vi "MetaServer.vi"(6 "Pause/Stop":cluster{"Exp Stop":bool, "ExpRun 2":bool}, 10 "File Paths":T1={"Local Save Path"=path "\\\\smbhome.uscs.susx.ac.uk\\cv222/Desktop/data", "Newton Save Path"=path "Z:/#Projects/Entanglement/data", "File Name"="test", "LocalSave"=TRUE}, 11 "Compiler Settings":T2={"Python Path"=path "", "Main File"="makesequence.py", "Meta File"="makesequence.py", "Aux File"="makesequence.py"}) -> ()   [LabVIEW 2017]
uses:
  PulseCompiler/CompilerSettings.ctl
  controls/FilePaths.ctl
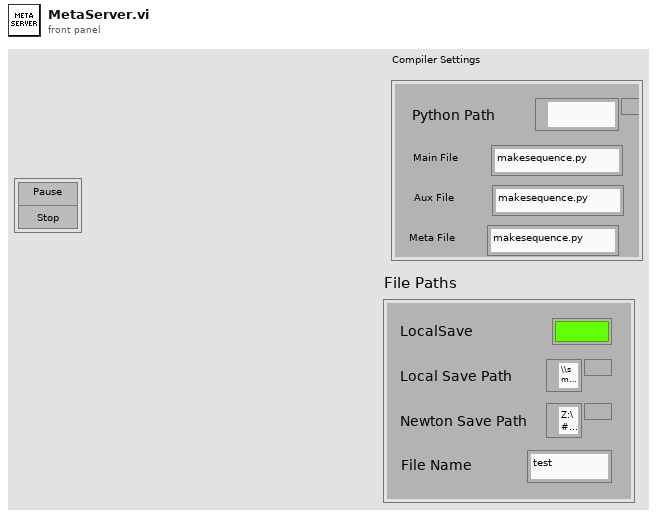
[diagram p1: front panel]
types:
  T1 = typedef "FilePaths.ctl" = cluster{"Local Save Path":path, "Newton Save Path":path, "File Name":string, "LocalSave":bool}
  T2 = typedef "CompilerSettings.ctl" = cluster{"Python Path":path, "Main File":string, "Meta File":string, "Aux File":string}
  T3 = cluster{"command":string, "steps":i32, "runs":i32}[]
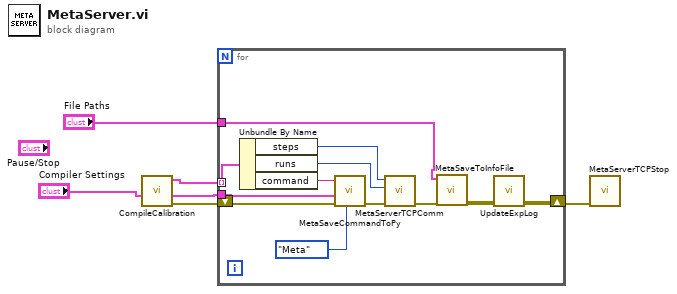
[diagram p0: block diagram]
diagram:
  n1 = call "CompileCalibration.vi"("Compiler Settings"="Compiler Settings") -> ("error out"=w5:errorcluster, "Compiler Settings 2"=w4:T2, "Exp out"=w6:T3)  [unwired: 8 in]
  n2 = for {
    tunnel: w6 -> [w18] mode=indexing
    tunnel: w4 -> [w14]
    shift-right: [w7] -> w2
    shift-left: w5 -> [w15]
    tunnel: "File Paths" -> [w11]
    n3 = Unbundle By Name(w18) -> ("steps"=w13:i32, "runs"=w12:i32, "command"=w17:string)
    n4 = call "MetaSaveCommandToPy.vi"("MetaorMain"=enum16{"Meta", "Main"}."Meta", "error in"=w15, "Compiler Settings In"=w14, "command"=w17) -> ("error out"=w10:errorcluster)  [unwired: 6 in, 1 out]
    n5 = call "MetaServerTCPComm.vi"("error in (no error)"=w10, "runs"=w12, "steps"=w13) -> ("error out"=w9:errorcluster)  [unwired: 8 in]
    n6 = call "MetaSaveToInfoFile.vi"("error in (no error)"=w9, "File Paths"=w11) -> ("error out"=w8:errorcluster)  [unwired: 9 in]
    n7 = call "UpdateExpLog.vi"("error in (no error)"=w8) -> ("error out"=w7:errorcluster)  [unwired: 10 in]
  }
  n8 = call "MetaServerTCPStop.vi"("error in (no error)"=w2) -> ()  [unwired: 10 in, 1 out]
